vi "SPC_read_gap_time.vi"(8 "Error In":errorcluster, 10 "Module No":i16 min=0 max=7 step=1, 11 "DLL Path":path) -> (0 "Error Out":errorcluster, 2 "Module No":i16, 3 "DLL Path":path, 4 "Time Value":sgl format="%.2f")   [LabVIEW 2023]
doc: "The procedure is used to read the gap time that can occur during a measurement with the sequencer of SPC6x0/130/150/131 modules. The variable ‘time’ should be set to the last gap time in ms on the SPC module specified by ‘mod_no’.\n\ninfo@becker-hickl.com"
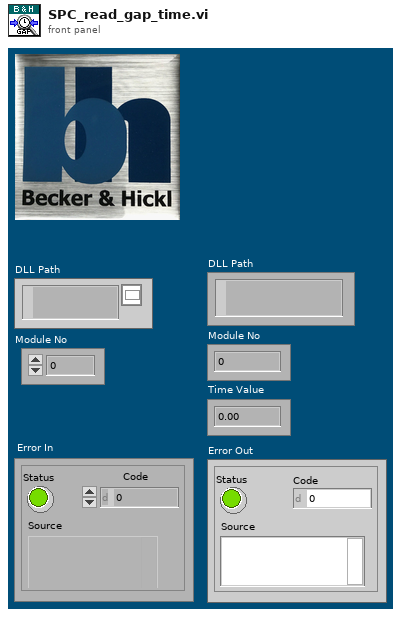
[diagram p1: front panel]
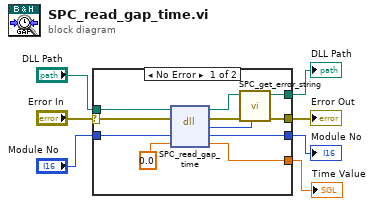
[diagram p0: block diagram]
diagram:
  n1 = case shown="No Error" "Error In" {
    selector: "Error In" -> [w18 w20]
    tunnel: "DLL Path" -> [w17 w21]
    tunnel: [w12 w21] -> w5
    tunnel: [w16 w20] -> w4
    tunnel: [w14 w19] -> w3
    tunnel: "Module No" -> [w10 w19]
    tunnel: [w8 _] -> w1
    frame No Error {
      n2 = dll-call lib="D:/spcm/lib/lab_view/lv10.0/spcm32.dll" fn="SPC_read_gap_time"(path in=w17, error in=w18, "mod_no"=w10, "time"=sgl 0.0 ("Last Time Value")) -> (path out=w13:path, error out=w15:errorcluster, "return type"=w11:i16, "mod_no"=w14:i16, "time"=w8:sgl)  [unwired: 1 in]
      n3 = call "SPC_get_error_string.vi"("ErrorID"=w11, "Error In"=w15, "DLL Path"=w13) -> ("Error Out"=w16:errorcluster, "DLL Path"=w12:path)  [unwired: 6 in, 1 out]
    }
    frame Error {
    }
  }
  "DLL Path" <- w5
  "Error Out" <- w4
  "Module No" <- w3
  "Time Value" <- w1
